vi "Plane_Enhancement.vi"() -> ()   [LabVIEW 2013]
uses:
  <vilib>/Analysis/Matrix/Numeric/Conversions/Array To Matrix - RA2.vi
  <vilib>/Analysis/Matrix/Numeric/Conversions/Matrix To Array - RM.vi
  <vilib>/vision/NI_Vision_Development_Module.lvlib
  <vilib>/Analysis/Matrix/NI_Matrix.lvlib
panel:
  in  "Numeric":dbl
  in  "Color Mode":u16(ring) items=["RGB", "HSL", "HSV", "HSI"]
  in  "Path":path
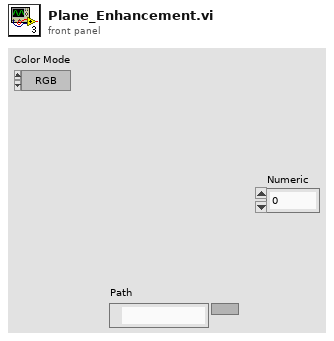
[diagram p1: front panel]
types:
  T1 = typedef "Image Type" = u32
  T2 = typedef "IMAQ Image.ctl" = refnum<image>
  T3 = typedef "NI_Matrix.lvlib/RealMatrix.ctl" = dbl[][]
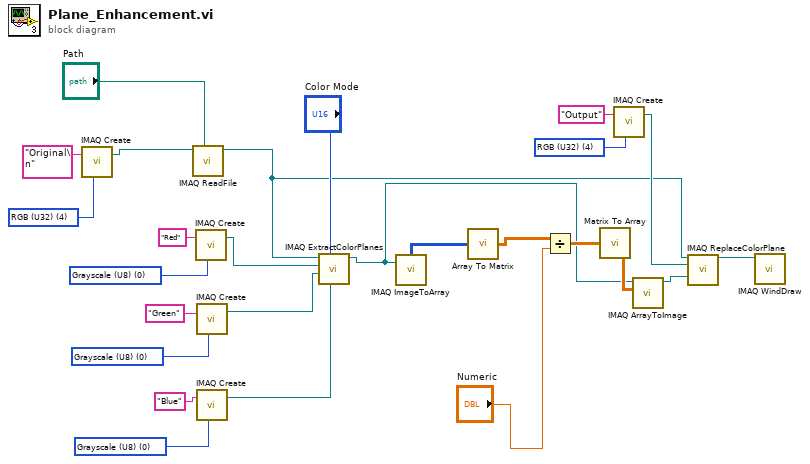
[diagram p0: block diagram]
diagram:
  w6 = T1 4 items=["Grayscale (U8)", "Grayscale (I16)", "Grayscale (SGL)", "Complex (CSG)", "RGB (U32)", "HSL (U32)", "RGB (U64)", "Grayscale (U16)"] ("Image Type")
  w17 = T1 0 items=["Grayscale (U8)", "Grayscale (I16)", "Grayscale (SGL)", "Complex (CSG)", "RGB (U32)", "HSL (U32)", "RGB (U64)", "Grayscale (U16)"] ("Image Type")
  w18 = T1 0 items=["Grayscale (U8)", "Grayscale (I16)", "Grayscale (SGL)", "Complex (CSG)", "RGB (U32)", "HSL (U32)", "RGB (U64)", "Grayscale (U16)"] ("Image Type")
  w19 = T1 0 items=["Grayscale (U8)", "Grayscale (I16)", "Grayscale (SGL)", "Complex (CSG)", "RGB (U32)", "HSL (U32)", "RGB (U64)", "Grayscale (U16)"] ("Image Type")
  w20 = T1 4 items=["Grayscale (U8)", "Grayscale (I16)", "Grayscale (SGL)", "Complex (CSG)", "RGB (U32)", "HSL (U32)", "RGB (U64)", "Grayscale (U16)"] ("Image Type")
  n1 = call "IMAQ Create"("Image Name"="Original\n", "Image Type"=w20) -> ("New Image"=w22:T2)  [unwired: 3 in, 1 out]
  n2 = call "IMAQ ReadFile"("File Path"="Path", "Image"=w22) -> ("Image Out"=w3:T2)  [unwired: 5 in, 4 out]
  n3 = call "IMAQ Create"("Image Name"="Red", "Image Type"=w19) -> ("New Image"=w16:T2)  [unwired: 3 in, 1 out]
  n4 = call "IMAQ Create"("Image Name"="Green", "Image Type"=w18) -> ("New Image"=w15:T2)  [unwired: 3 in, 1 out]
  n5 = call "IMAQ Create"("Image Name"="Blue", "Image Type"=w17) -> ("New Image"=w13:T2)  [unwired: 3 in, 1 out]
  n6 = call "IMAQ ExtractColorPlanes"("Blue or Luma or Val or Inten Plane"=w13, "Color Mode"="Color Mode", "Green or Sat Plane"=w15, "Red or Hue Plane"=w16, "Image Src"=w3) -> ("Red or Hue Plane out"=w8:T2)  [unwired: 3 in, 3 out]
  n7 = call "IMAQ ImageToArray"("Image"=w8) -> ("Image Pixels (U8)"=w12:u8[][])  [unwired: 3 in, 4 out]
  n8 = call-poly <vilib>:"Array To Matrix.vi"("Real 2D Array"=w12) -> ("Real Matrix"=w11:T3)
  n9 = Divide(x=w11, y="Numeric") -> (x/y=w10:T3)
  n10 = call-poly <vilib>:"Matrix To Array.vi"("Real Matrix"=w10) -> ("Real 2D Array"=w9:dbl[][])
  n11 = call "IMAQ Create"("Image Name"="Output", "Image Type"=w6) -> ("New Image"=w4:T2)  [unwired: 3 in, 1 out]
  n12 = call "IMAQ ArrayToImage"("Image Pixels (U8)"=w9, "Image"=w8) -> ("Image Out"=w5:T2)  [unwired: 8 in, 1 out]
  n13 = call "IMAQ ReplaceColorPlane"("Image Src"=w3, "Image Dst"=w4, "Green or Sat Plane"=w5) -> ("Image Dst Out"=w2:T2)  [unwired: 11 in, 1 out]
  n14 = call "IMAQ WindDraw"("Image"=w2) -> ()  [unwired: 9 in, 2 out]
